vi "Get Hierarchy.vi"(8 "error in (no error)":errorcluster, 11 "Security in":refnum<class "Security.lvclass">) -> (0 "error out":errorcluster, 2 "Hierarchy":T1, 3 "Security out":refnum<class "Security.lvclass">)   [LabVIEW 2020, in "HTTP Server.lvlib" / "Security.lvclass"]
uses:
  Security.lvclass
  Hierarchy.ctl
  Security.lvclass/Security.ctl
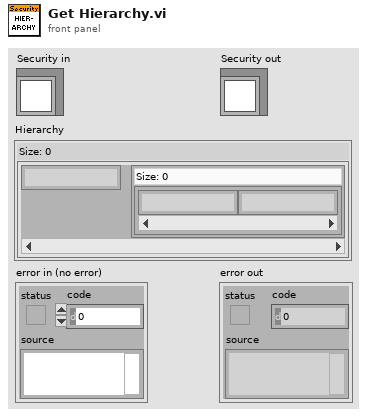
[diagram p1: front panel]
types:
  T1 = typedef "HTTP Server.lvlib/Security.lvclass/Hierarchy.ctl" = map{string, set{string}}
  T2 = typedef "HTTP Server.lvlib/Security.lvclass/Ref Data.ctl" = cluster{"Hierarchy":T1}
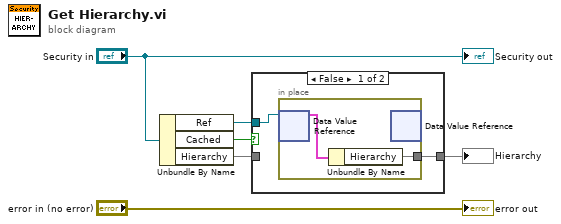
[diagram p0: block diagram]
diagram:
  n1 = Unbundle By Name("Security in") -> ("Ref"=w3:refnum<data-value>, "Cached"=w4:bool, "Hierarchy"=w2:T1)
  n2 = case shown="False" w4 {
    tunnel: w3 -> [w8 _]
    tunnel: w2 -> [_ w11]
    tunnel: [w7 w11] -> w1
    frame False {
      n3 = in-place {
        in-place-border: [w9] -> w7
        n4 = in-place-dvr #1(w8) -> (w10:T2)  [unwired: 1 out]
        n5 = Unbundle By Name(w10) -> ("Hierarchy"=w9:T1)
        n6 = in-place-dvr #1() -> ()  [unwired: 1 in, 2 out]
      }
    }
    frame True {
    }
  }
  "Hierarchy" <- w1
  "error out" <- "error in (no error)"
  "Security out" <- "Security in"
